vi "fgv_950_cmd_sort.vi"() -> ()   [LabVIEW 2019]
uses:
  cmd_dl950_sort.ctl
panel:
  in  "range(+5)":dbl
  in  "range(-5)":dbl
  in  "high":i16=4
  in  "middle":i16=4
  in  "low":i16=4
  in  "cmd":T1
  in  "ch":i16=4
  out "resulting string":string
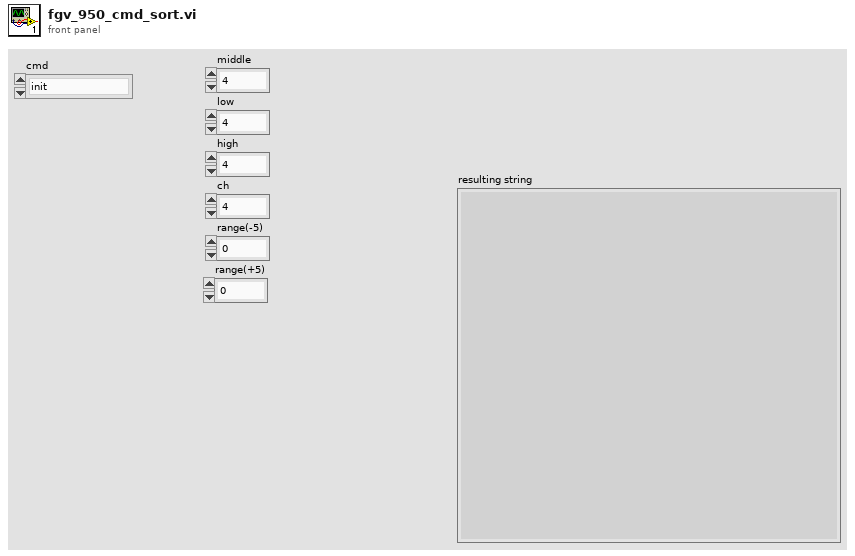
[diagram p1: front panel]
types:
  T1 = typedef "cmd_dl950_sort.ctl" = enum16{"init", "item off", "set_check_ini_on", "meas_check_ini", "set_cap_on", "meas_cap", "set_res_on", "meas_res", "set_b1_on", "meas_b1", "set_b2_on", "meas_b2", "set_b3_on", "meas_b3", "idle"}
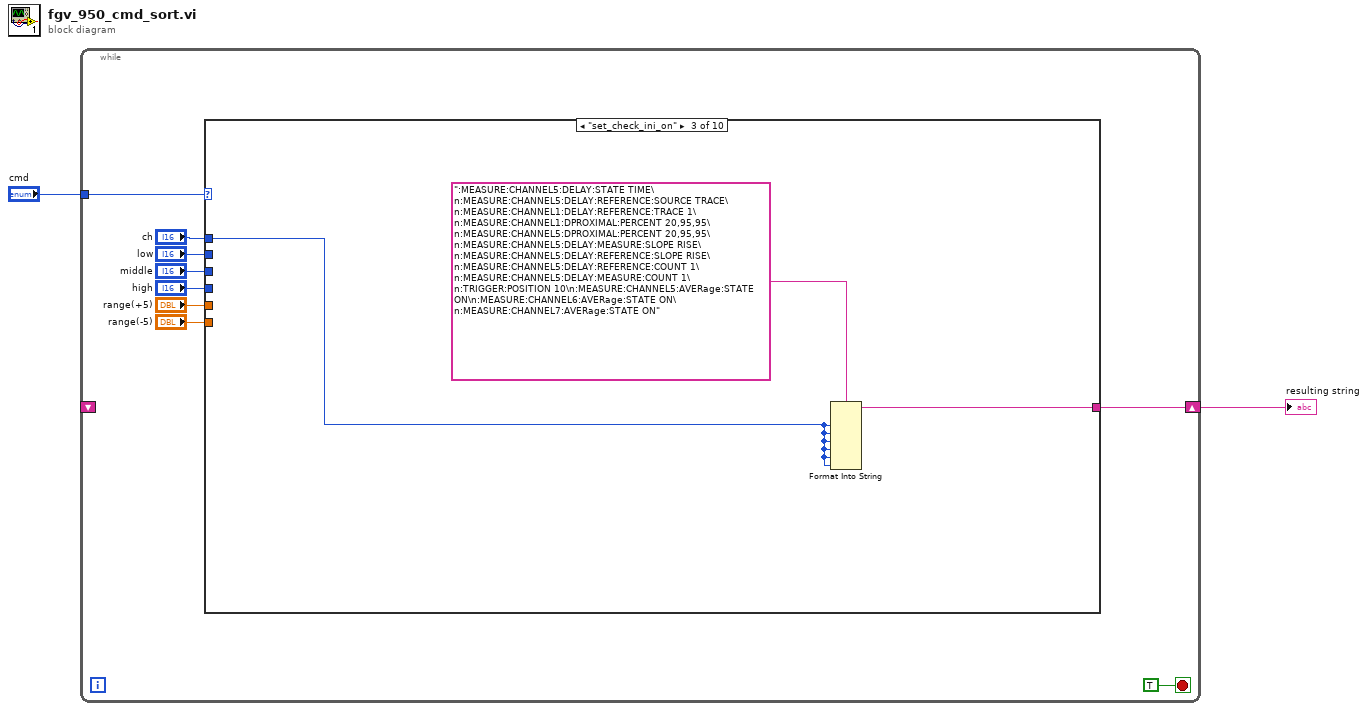
[diagram p0: block diagram]
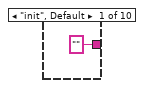
[diagram p2: hidden frame]
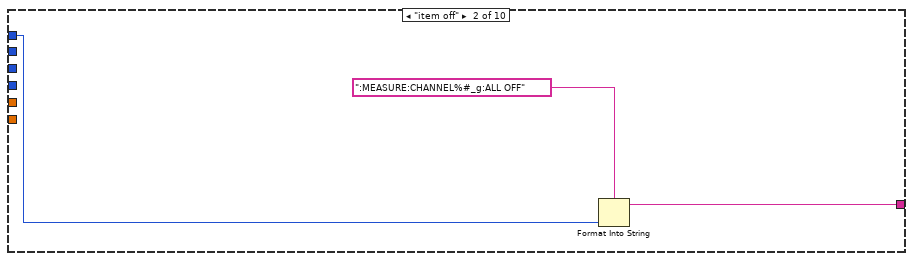
[diagram p3: hidden frame]
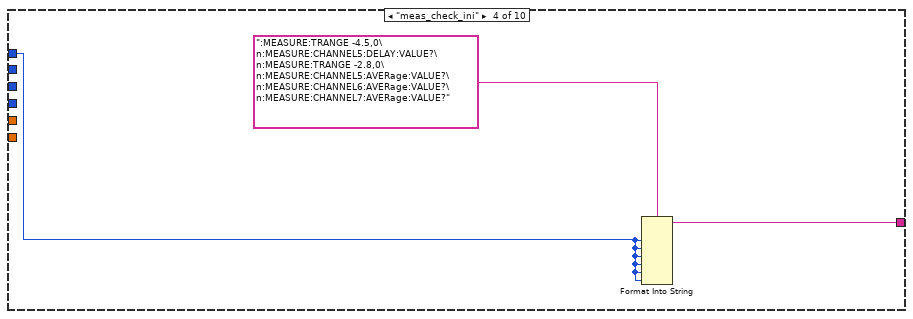
[diagram p4: hidden frame]
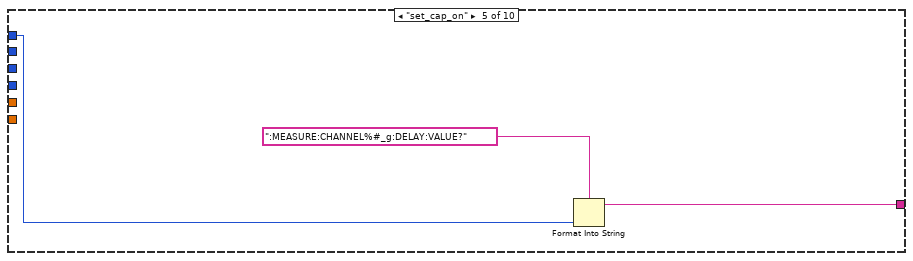
[diagram p5: hidden frame]
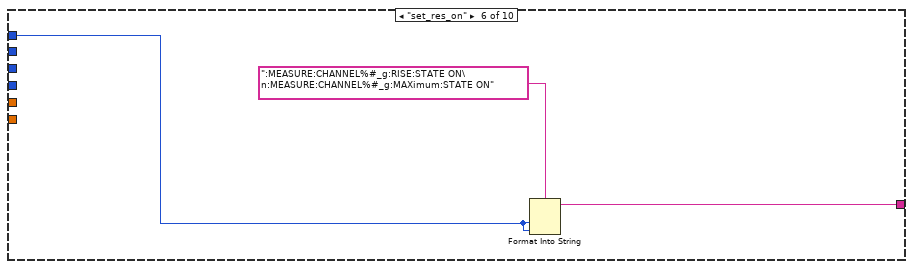
[diagram p6: hidden frame]
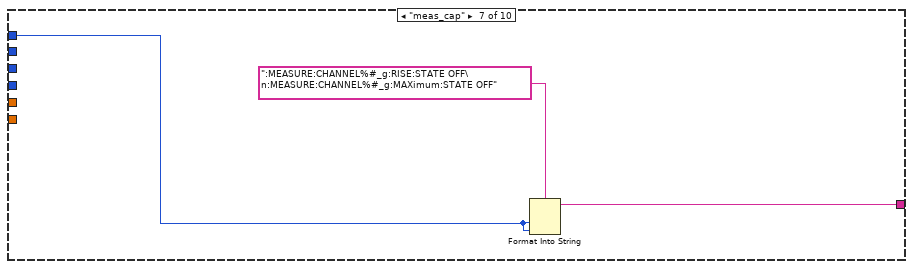
[diagram p7: hidden frame]
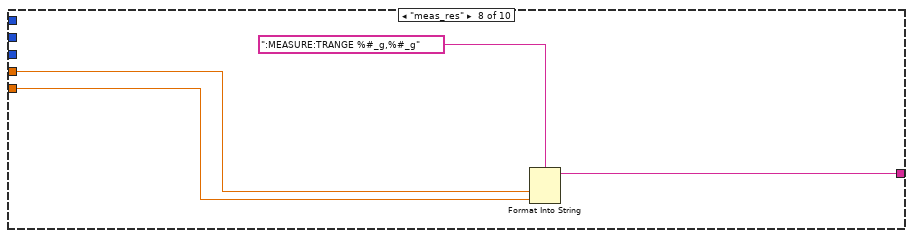
[diagram p8: hidden frame]
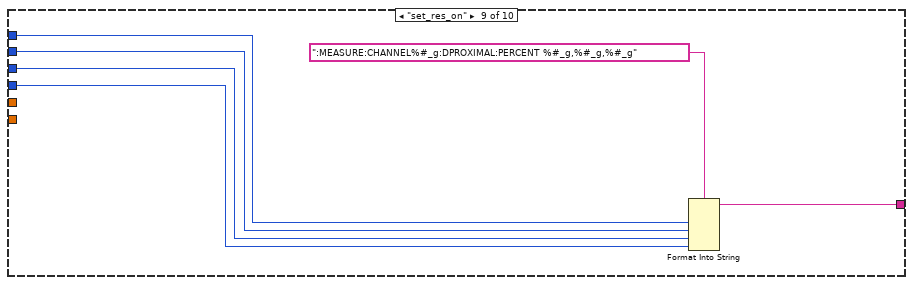
[diagram p9: hidden frame]
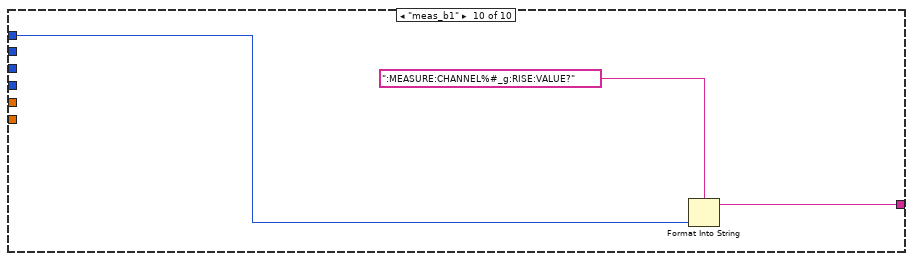
[diagram p10: hidden frame]
diagram:
  n1 = while {
    tunnel: "cmd" -> [w9]
    shift-right: [w10] -> w2
    shift-left: _ -> [_]
    stop <- TRUE stop-if-true
    n2 = case shown="\"set_check_ini_on\"" w9 {
      tunnel: ["" w14 w17 w19 w23 w25 w28 w33 w39 w43] -> w10
      tunnel: "ch" -> [_ w13 w16 w20 w22 w26 w29 _ w35 w42]
      tunnel: "low" -> [_ _ _ _ _ _ _ _ w38 _]
      tunnel: "middle" -> [_ _ _ _ _ _ _ _ w37 _]
      tunnel: "high" -> [_ _ _ _ _ _ _ _ w36 _]
      tunnel: "range(+5)" -> [_ _ _ _ _ _ _ w32 _ _]
      tunnel: "range(-5)" -> [_ _ _ _ _ _ _ w31 _ _]
      frame "init", Default {
      }
      frame "item off" {
        n3 = Format Into String(format string=":MEASURE:CHANNEL%#_g:ALL OFF", w13) -> (resulting string=w14:string)  [unwired: 2 in, 1 out]
      }
      frame "set_check_ini_on" {
        n4 = Format Into String(format string=":MEASURE:CHANNEL5:DELAY:STATE TIME\n:MEASURE:CHANNEL5:DELAY:REFERENCE:SOURCE TRACE\n:MEASURE:CHANNEL1:DELAY:REFERENCE:TRACE 1\n:MEASURE:CHANNEL1:DPROXIMAL:PERCENT 20,95,95\n:MEASURE:CHANNEL5:DPROXIMAL:PERCENT 20,95,95\n:MEASURE:CHANNEL5:DELAY:MEASURE:SLOPE RISE\n:MEASURE:CHANNEL5:DELAY:REFERENCE:SLOPE RISE\n:MEASURE:CHANNEL5:DELAY:REFERENCE:COUNT 1\n:MEASURE:CHANNEL5:DELAY:MEASURE:COUNT 1\n:TRIGGER:POSITION 10\n:MEASURE:CHANNEL5:AVERage:STATE ON\n:MEASURE:CHANNEL6:AVERage:STATE ON\n:MEASURE:CHANNEL7:AVERage:STATE ON", w16, w16, w16, w16, w16, w16) -> (resulting string=w17:string)  [unwired: 2 in, 1 out]
      }
      frame "meas_check_ini" {
        n5 = Format Into String(format string=":MEASURE:TRANGE -4.5,0\n:MEASURE:CHANNEL5:DELAY:VALUE?\n:MEASURE:TRANGE -2.8,0\n:MEASURE:CHANNEL5:AVERage:VALUE?\n:MEASURE:CHANNEL6:AVERage:VALUE?\n:MEASURE:CHANNEL7:AVERage:VALUE?", w20, w20, w20, w20, w20, w20) -> (resulting string=w19:string)  [unwired: 2 in, 1 out]
      }
      frame "set_cap_on" {
        n6 = Format Into String(format string=":MEASURE:CHANNEL%#_g:DELAY:VALUE?", w22) -> (resulting string=w23:string)  [unwired: 2 in, 1 out]
      }
      frame "set_res_on" {
        n7 = Format Into String(format string=":MEASURE:CHANNEL%#_g:RISE:STATE ON\n:MEASURE:CHANNEL%#_g:MAXimum:STATE ON", w26, w26) -> (resulting string=w25:string)  [unwired: 2 in, 1 out]
      }
      frame "meas_cap" {
        n8 = Format Into String(format string=":MEASURE:CHANNEL%#_g:RISE:STATE OFF\n:MEASURE:CHANNEL%#_g:MAXimum:STATE OFF", w29, w29) -> (resulting string=w28:string)  [unwired: 2 in, 1 out]
      }
      frame "meas_res" {
        n9 = Format Into String(format string=":MEASURE:TRANGE %#_g,%#_g", w32, w31) -> (resulting string=w33:string)  [unwired: 2 in, 1 out]
      }
      frame "set_res_on" {
        n10 = Format Into String(format string=":MEASURE:CHANNEL%#_g:DPROXIMAL:PERCENT %#_g,%#_g,%#_g", w35, w38, w37, w36) -> (resulting string=w39:string)  [unwired: 2 in, 1 out]
      }
      frame "meas_b1" {
        n11 = Format Into String(format string=":MEASURE:CHANNEL%#_g:RISE:VALUE?", w42) -> (resulting string=w43:string)  [unwired: 2 in, 1 out]
      }
    }
  }
  "resulting string" <- w2
